vi "raw queue to image queue_MD.vi"() -> ()   [LabVIEW 2012]
uses:
  <vilib>/Utility/VariantDataType/Type.ctl
  GFG/GFGnumericGet.vi
  GFG/GFGbooleanGet.vi
  GFG/GFG library.lvlib
  <vilib>/Utility/VariantDataType/VariantType.lvlib
panel:
  out "error out 4":errorcluster
  out "error out 3":errorcluster
  out "error out 2":errorcluster
  out "# elements in raw queue":i32
  out "error out":errorcluster
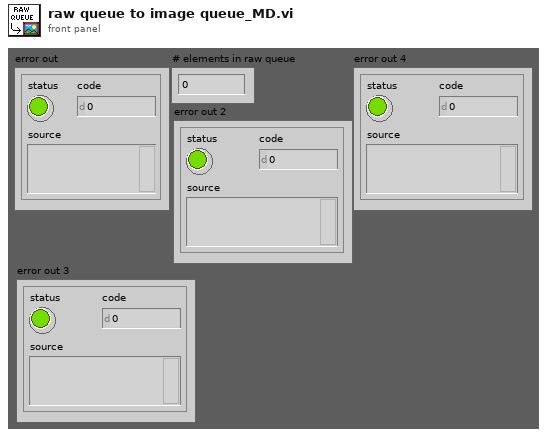
[diagram p1: front panel]
types:
  T1 = cluster{"NewVal":bool, "Event Registration Refnum":refnum<event-registration>}
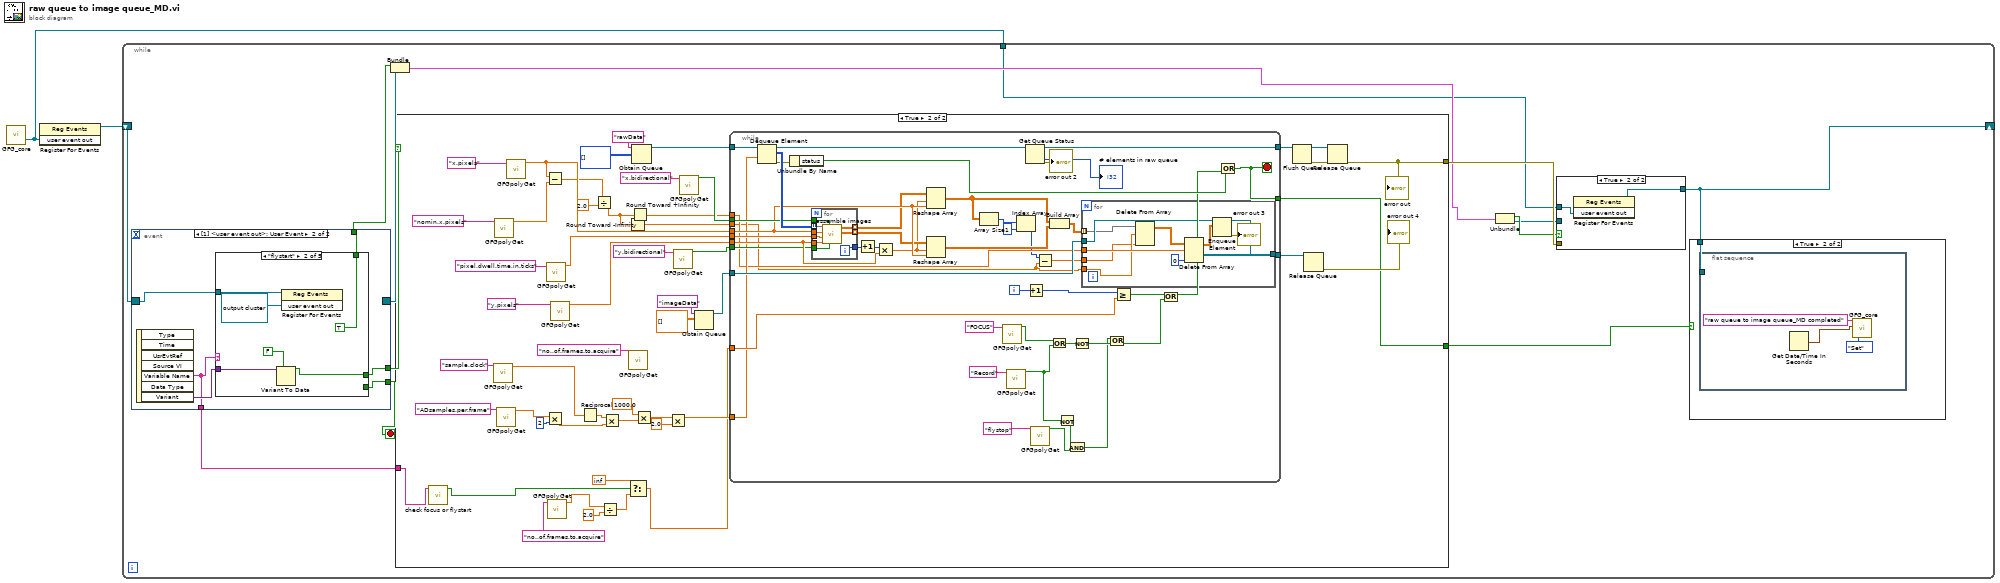
[diagram p0: block diagram]
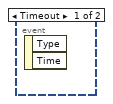
[diagram p4: hidden frame]
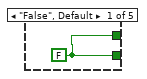
[diagram p5: hidden frame]
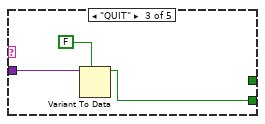
[diagram p6: hidden frame]
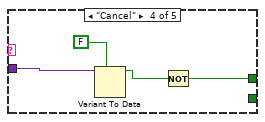
[diagram p7: hidden frame]
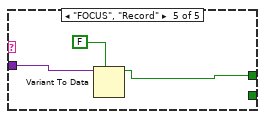
[diagram p8: hidden frame]
diagram:
  n1 = call "GFG_core.vi"() -> ("user event out"=w1:refnum<user-event>)  [unwired: 13 in, 6 out]
  n2 = register-events(w1) -> (reference out=w2:refnum<event-registration>)  [unwired: 2 in, 1 out]
  n3 = while {
    shift-right: [w4] -> _
    shift-left: w2 -> [w15]
    tunnel: w1 -> [w6]
    stop <- w14 stop-if-true
    n4 = event shown="[1] <user event out>: User Event" {
      selector: w15 -> [_ w25]
      dyn-events: [_ _] -> w11
      timeout: _ -> [_ _]
      tunnel: [_ w28] -> w13
      tunnel: [_ w27] -> w14
      tunnel: [_ w24] -> w12
      tunnel: [_ w23] -> w5
      event Timeout {
        n5 = event-data() -> ()  [unwired: 1 in, 2 out]
      }
      event User Event {
        n6 = event-data() -> ("Variable Name"=w23:string, "Variant"=w26:variant)  [unwired: 1 in, 5 out]
        n7 = case shown="\"flystart\"" w23 {
          tunnel: [w29 w33 _ w39 w43] -> w28
          tunnel: [w29 _ w36 _ _] -> w27
          tunnel: w26 -> [_ w34 w38 w41 w44]
          tunnel: w25 -> [_ w31 _ _ _]
          tunnel: [_ TRUE ("NewVal") _ _ _] -> w24
          frame "False", Default {
            w29 = FALSE ("NewVal")
          }
          frame "flystart" {
            n8 = Variant To Data(type=FALSE ("NewVal"), Variant=w34) -> (data=w33:bool)  [unwired: 1 in, 1 out]
            n9 = register-events(reference=w31, refnum<user-event> refnum ("user event out")) -> ()  [unwired: 1 in, 2 out]
          }
          frame "QUIT" {
            n10 = Variant To Data(type=FALSE ("NewVal"), Variant=w38) -> (data=w36:bool)  [unwired: 1 in, 1 out]
          }
          frame "Cancel" {
            n11 = Variant To Data(type=FALSE ("NewVal"), Variant=w41) -> (data=w40:bool)  [unwired: 1 in, 1 out]
            n12 = Not(x=w40) -> (.not. x?=w39:bool)
          }
          frame "FOCUS", "Record" {
            n13 = Variant To Data(type=FALSE ("NewVal"), Variant=w44) -> (data=w43:bool)  [unwired: 1 in, 1 out]
          }
        }
      }
    }
    n14 = Bundle("NewVal"=w12, "Event Registration Refnum"=w11) -> (w9:T1)  [unwired: 1 in]
    n15 = case shown="True" w13 {
      tunnel: [_ w54] -> w10
      tunnel: w5 -> [_ w48]
      tunnel: [_ w46] -> w3
      frame False {
      }
      frame True {
        n16 = call "check focus or flystart.vi"("x"=w48) -> ("x .or. y?"=w47:bool)  [unwired: 10 in]
        n17 = call-poly "GFGpolyGet.vi"("Variable Name in"="sample.clock" ("Tag in")) -> ("Numeric"=w69:dbl)  [unwired: 9 in, 1 out]
        n18 = call-poly "GFGpolyGet.vi"("Variable Name in"="nomin.x.pixels" ("Tag in")) -> ("Numeric"=w62:dbl)  [unwired: 9 in, 1 out]
        n19 = call-poly "GFGpolyGet.vi"("Variable Name in"="ADsamples.per.frame" ("Tag in")) -> ("Numeric"=w74:dbl)  [unwired: 9 in, 1 out]
        n20 = call-poly "GFGpolyGet.vi"("Variable Name in"="x.pixels" ("Tag in")) -> ("Numeric"=w61:dbl)  [unwired: 9 in, 1 out]
        n21 = Subtract(x=w61, y=w62) -> (x-y=w60:dbl)
        n22 = Multiply(x=w74, y=i8 2) -> (x*y=w68:dbl)
        n23 = call-poly "GFGpolyGet.vi"("Variable Name in"="pixel.dwell.time.in.ticks" ("Tag in")) -> ("Numeric"=w86:dbl)  [unwired: 9 in, 1 out]
        n24 = call-poly "GFGpolyGet.vi"("Variable Name in"="no..of.frames.to.acquire" ("Tag in")) -> ("Numeric"=w51:dbl)  [unwired: 9 in, 1 out]
        n25 = call-poly "GFGpolyGet.vi"("Variable Name in"="y.pixels" ("Tag in")) -> ("Numeric"=w79:dbl)  [unwired: 9 in, 1 out]
        n26 = Reciprocal(x=w69) -> (1/x=w73:dbl)
        n27 = Divide(x=w60, y=2.0) -> (x/y=w57:dbl)
        n28 = Divide(x=w51, y=2.0) -> (x/y=w50:dbl)
        n29 = Multiply(x=w73, y=w68) -> (x*y=w72:dbl)
        n30 = Round Toward -Infinity(1:w57) -> (0:w56:dbl)
        n31 = call-poly "GFGpolyGet.vi"("Variable Name in"="no..of.frames.to.acquire" ("Tag in")) -> ()  [unwired: 9 in, 2 out]
        n32 = Select(t=inf, s=w47, f=w50) -> (s? t:f=w49:dbl)
        n33 = Round Toward +Infinity(x=w57) -> (ceil(x): smallest int >= x=w58:dbl)
        n34 = Obtain Queue(name (unnamed)="rawData", element data type=i16[][] [] ("-x")) -> (queue out=w91:refnum<queue>)  [unwired: 3 in, 2 out]
        n35 = Multiply(x=1000.0, y=w72) -> (x*y=w66:dbl)
        n36 = Multiply(x=w66, y=2.0) -> (x*y=w65:dbl)
        n37 = call-poly "GFGpolyGet.vi"("Variable Name in"="y.bidirectional") -> ("Boolean"=w83:bool)  [unwired: 10 in]
        n38 = call-poly "GFGpolyGet.vi"("Variable Name in"="x.bidirectional") -> ("Boolean"=w81:bool)  [unwired: 10 in]
        n39 = Obtain Queue(name (unnamed)="imageData", element data type=dbl[][] [] ("y backward image")) -> (queue out=w93:refnum<queue>)  [unwired: 3 in, 2 out]
        n40 = while {
          tunnel: w91 -> [w129]
          tunnel: [w122] -> w89
          tunnel: w93 -> [w143]
          tunnel: [w142] -> w92
          tunnel: w61 -> [w136]
          tunnel: w79 -> [w141]
          tunnel: w86 -> [w140]
          tunnel: w83 -> [w138]
          tunnel: w81 -> [w137]
          tunnel: w49 -> [w134]
          tunnel: w65 -> [w130]
          tunnel: w58 -> [w112]
          tunnel: w56 -> [w107]
          tunnel: [w103] -> w46
          i -> [w131]
          stop <- w103 stop-if-true
          n41 = Dequeue Element(queue=w129, timeout in ms (-1)=w130) -> (queue out=w123:refnum<queue>, element=w139:i16[][], error out=w133:errorcluster)  [unwired: 1 in, 1 out]
          n42 = Unbundle By Name(w133) -> ("status"=w135:bool)
          n43 = for {
            tunnel: w139 -> [w149] mode=indexing
            tunnel: w140 -> [w151]
            tunnel: w136 -> [w150]
            tunnel: w141 -> [w152]
            tunnel: [w148] -> w118 mode=indexing
            tunnel: [w147] -> w117 mode=indexing
            tunnel: w138 -> [w145]
            tunnel: w137 -> [w146]
            tunnel: [w144] -> w114
            i -> [w144]
            n44 = call "assemble images.vi"("bidi_y"=w145, "bidi_x"=w146, "y pixels"=w152, "bin factor"=w151, "x pixels"=w150, "raw data in (negative 11 bit data)"=w149) -> ("second image"=w147:dbl[][], "first image"=w148:dbl[][])  [unwired: 4 in]
          }
          n45 = Increment(x=w114) -> (x+1=w113:i32)
          n46 = Multiply(x=w113, y=w141) -> (x*y=w116:dbl)
          n47 = Reshape Array(w118, w116, w136) -> (w111:dbl[][])
          n48 = Reshape Array(w117, w116, w136) -> (w115:dbl[][])
          n49 = Array Size(array=w111) -> (size(s)=w110:i32[])
          n50 = call-poly "GFGpolyGet.vi"("Variable Name in"="FOCUS") -> ("Boolean"=w126:bool)  [unwired: 10 in]
          n51 = call-poly "GFGpolyGet.vi"("Variable Name in"="Record") -> ("Boolean"=w99:bool)  [unwired: 10 in]
          n52 = Index Array(array=w110, index=1) -> (element=w108:i32)
          n53 = Get Queue Status(queue=w123) -> (queue out=w122:refnum<queue>, error out=→"error out 2":errorcluster, # elements in queue=→"# elements in raw queue":i32)  [unwired: 2 in, 5 out]
          n54 = Increment(x=w131) -> (x+1=w120:i32)
          n55 = call-poly "GFGpolyGet.vi"("Variable Name in"="flystop") -> ("Boolean"=w100:bool)  [unwired: 10 in]
          n56 = Subtract(x=w108, y=w107) -> (x-y=w106:dbl)
          n57 = Build Array(w111, w115) -> (w119:dbl[][][])
          n58 = Or(x=w126, y=w99) -> (x .or. y?=w124:bool)
          n59 = Not(x=w99) -> (.not. x?=w101:bool)
          n60 = And(x=w101, y=w100) -> (x .and. y?=w97:bool)
          n61 = Not(x=w124) -> (.not. x?=w104:bool)
          n62 = for {
            tunnel: w119 -> [w155] mode=indexing
            tunnel: w143 -> [w162]
            tunnel: [w161] -> w142
            tunnel: w112 -> [w160]
            tunnel: w107 -> [w158]
            tunnel: w106 -> [w157]
            n63 = Delete From Array(array=w155, length=w158, index (col)=w157) -> (array with subset deleted=w156:dbl[][])  [unwired: 1 in, 1 out]
            n64 = Delete From Array(array=w156, length=w160, index (col)=0 ("disabled index (col)")) -> (array with subset deleted=w154:dbl[][])  [unwired: 1 in, 1 out]
            n65 = Enqueue Element(queue=w162, element=w154) -> (queue out=w161:refnum<queue>, error out=→"error out 3":errorcluster)  [unwired: 2 in, 1 out]
          }
          n66 = Or(x=w97, y=w104) -> (x .or. y?=w98:bool)
          n67 = Greater Or Equal?(x=w120, y=w134) -> (x >= y?=w132:bool)
          n68 = Or(x=w132, y=w98) -> (x .or. y?=w125:bool)
          n69 = Or(x=w135, y=w125) -> (x .or. y?=w103:bool)
        }
        n70 = Flush Queue(queue=w89) -> (queue out=w88:refnum<queue>, error out=w77:errorcluster)  [unwired: 1 in, 1 out]
        n71 = Release Queue(queue=w92) -> (error out=→"error out 4":errorcluster)  [unwired: 2 in, 2 out]
        n72 = Release Queue(queue=w88, error in (no error)=w77) -> (error out=w54:errorcluster)  [unwired: 1 in, 2 out]
        "error out" <- w54
      }
    }
    n73 = Unbundle(w9) -> ("NewVal"=w8:bool, "Event Registration Refnum"=w7:refnum<event-registration>)
    n74 = case shown="True" w8 {
      tunnel: [w20 w22] -> w4
      tunnel: w10 -> [_ _]
      tunnel: w7 -> [w20 _]
      tunnel: w6 -> [_ w21]
      frame False {
      }
      frame True {
        n75 = register-events(w21) -> (reference out=w22:refnum<event-registration>)  [unwired: 2 in, 1 out]
      }
    }
    n76 = case shown="True" w3 {
      tunnel: w4 -> [_ w16]
      frame False {
      }
      frame True {
        n77 = flat-sequence {
          tunnel: w16 -> [_]
          frame #0 {
            n78 = Get Date/Time In Seconds() -> (seconds since 1Jan1904=w17:timestamp)
            n79 = call "GFG_core.vi"("Variable Name in"="raw queue to image queue_MD completed", "Variant in"=w17, "Action"=enum16{"Init", "Set", "Get"}."Set") -> ()  [unwired: 10 in, 7 out]
          }
        }
      }
    }
  }
